vi "setSerializedData.vi"(0 "reference":refnum<class "CallNode.lvclass">, 1 "parent":refnum<class "AbstractNode.lvclass">, 2 "children":refnum<class "AbstractNode.lvclass">[](array[class]), 3 "xmlOut":string, 5 "error in (no error)":errorcluster) -> (14 "reference out":refnum<class "CallNode.lvclass">, 19 "error out":errorcluster)   [LabVIEW 2014, in "CallNode.lvclass"]
doc: "setSerializedData"
uses:
  <resource>/Framework/Providers/Open_GDS/UML/CallNode_class/CallNode.lvclass
  <resource>/Framework/Providers/Open_GDS/UML/AbstractNode_class/AbstractNode.lvclass
  <resource>/Framework/Providers/Open_GDS/UML/General/Rectangle/Rectangle Rectangle2D.ctl
  <resource>/Framework/Providers/Open_GDS/UML/RectangularNode_class/RectangularNode.lvclass
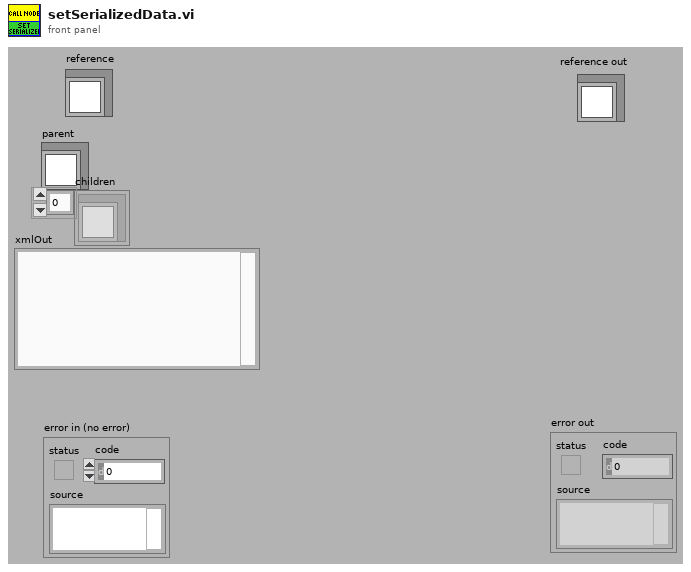
[diagram p1: front panel]
types:
  T1 = typedef "Rectangle Rectangle2D.ctl" = cluster{"x":dbl, "y":dbl, "width":dbl, "height":dbl}
  T2 = cluster{"Base class":cluster{"Base class":cluster{"parent":refnum<k1>, "children":refnum<k1>[]}, "bounds":T1}, "objectCallNodeRef":refnum<k1>, "signaled":bool, "openBottom":bool, "DEFAULT_WIDTH":i32, "DEFAULT_HEIGHT":i32, "CALL_YGAP":i32}
  T3 = typedef "RectangularNode.lvclass/ObjectAttributes.ctl" = cluster{"bounds":T1}
  T4 = typedef "AbstractNode.lvclass/ObjectAttributes.ctl" = cluster{"parent":refnum<class "AbstractNode.lvclass">, "children":refnum<class "AbstractNode.lvclass">[], "Hidden":bool}
  T5 = typedef "CallNode.lvclass/ObjectAttributes.ctl" = cluster{"objectCallNodeRef":refnum<class "AbstractNode.lvclass">, "signaled":bool, "openBottom":bool, "DEFAULT_WIDTH":i32, "DEFAULT_HEIGHT":i32, "CALL_YGAP":i32}
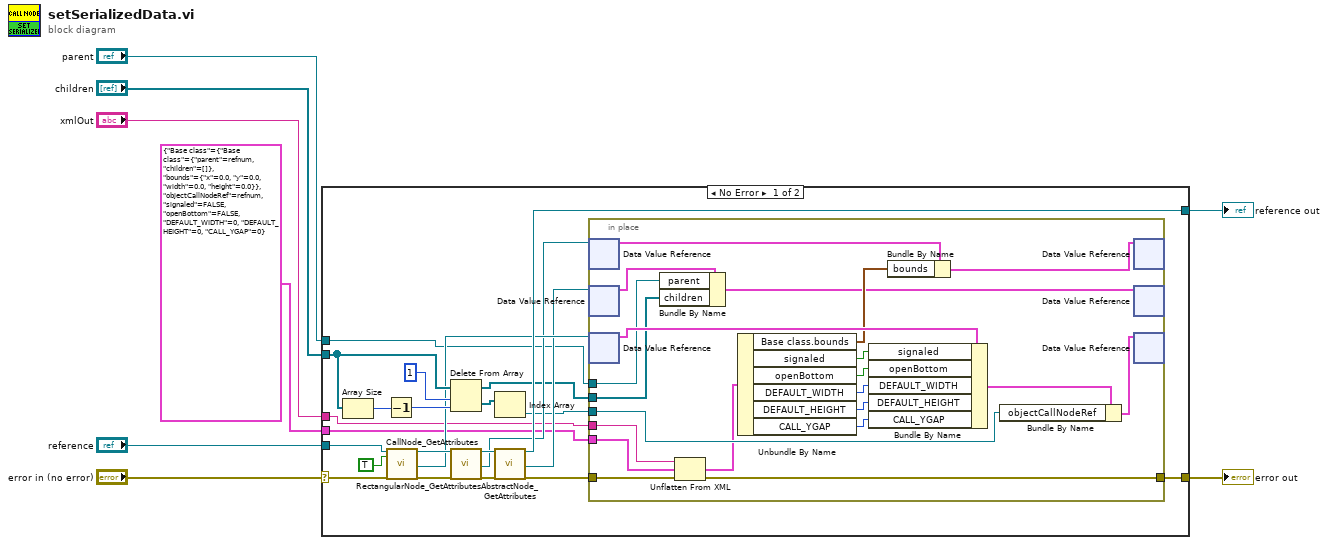
[diagram p0: block diagram]
diagram:
  n1 = case shown="No Error" "error in (no error)" {
    selector: "error in (no error)" -> [w30 w53]
    tunnel: "reference" -> [w31 w54]
    tunnel: [w29 w53] -> w6
    tunnel: [w28 w54] -> w5
    tunnel: "xmlOut" -> [w11 _]
    tunnel: "parent" -> [w10 _]
    tunnel: "children" -> [w24 _]
    tunnel: T2 {"Base class"={"Base class"={"parent"=refnum, "children"=[]}, "bounds"={"x"=0.0, "y"=0.0, "width"=0.0, "height"=0.0}}, "objectCallNodeRef"=refnum, "signaled"=FALSE, "openBottom"=FALSE, "DEFAULT_WIDTH"=0, "DEFAULT_HEIGHT"=0, "CALL_YGAP"=0} ("Attributes") -> [w12 _]
    frame No Error {
      n2 = Array Size(array=w24) -> (size(s)=w26:i32)
      n3 = Decrement(x=w26) -> (x-1=w27:i32)
      n4 = call <resource>:"CallNode_GetAttributes.vi"("reference in"=w31, "OnlyGetDvrReference(False)"=TRUE, "error in (no error)"=w30) -> ("reference out"=w21:refnum<class "CallNode.lvclass">, "DataRef"=w17:refnum<data-value>, "error out"=w20:errorcluster)  [unwired: 13 in, 1 out]
      n5 = Delete From Array(array=w24, length=1, index=w27) -> (deleted portion=w23:refnum<class "AbstractNode.lvclass">[], array with subset deleted=w9:refnum<class "AbstractNode.lvclass">[])
      n6 = call <resource>:"RectangularNode_GetAttributes.vi"("reference in"=w21, "error in (no error)"=w20) -> ("reference out"=w19:refnum<class "CallNode.lvclass">, "DataRef"=w16:refnum<data-value>, "error out"=w18:errorcluster)  [unwired: 14 in, 1 out]
      n7 = Index Array(array=w23) -> (element=w14:refnum<class "AbstractNode.lvclass">)  [unwired: 1 in]
      n8 = call <resource>:"AbstractNode_GetAttributes.vi"("reference in"=w19, "error in (no error)"=w18) -> ("reference out"=w28:refnum<class "CallNode.lvclass">, "DataRef"=w15:refnum<data-value>, "error out"=w13:errorcluster)  [unwired: 14 in, 1 out]
      n9 = in-place {
        in-place-border: w14 -> [w45]
        in-place-border: w13 -> [w41]
        in-place-border: w12 -> [w40]
        in-place-border: w11 -> [w39]
        in-place-border: [w38] -> w29
        in-place-border: w10 -> [w35]
        in-place-border: w9 -> [w34]
        n10 = in-place-dvr #1(w16) -> (w37:T3)  [unwired: 1 out]
        n11 = in-place-dvr #2(w15) -> (w36:T4)  [unwired: 1 out]
        n12 = in-place-dvr #3(w17) -> (w52:T5)  [unwired: 1 out]
        n13 = Bundle By Name(cluster=w36, "parent"=w35, "children"=w34) -> (w32:T4)
        n14 = Unflatten From XML(xml string=w39, type=w40, error in (no error)=w41) -> (value=w43:T2, error out=w38:errorcluster)
        n15 = Unbundle By Name(w43) -> ("Base class.bounds"=w42:T1, "signaled"=w51:bool, "openBottom"=w50:bool, "DEFAULT_WIDTH"=w49:i32, "DEFAULT_HEIGHT"=w48:i32, "CALL_YGAP"=w47:i32)
        n16 = Bundle By Name(cluster=w52, "signaled"=w51, "openBottom"=w50, "DEFAULT_WIDTH"=w49, "DEFAULT_HEIGHT"=w48, "CALL_YGAP"=w47) -> (w46:T5)
        n17 = Bundle By Name(cluster=w37, "bounds"=w42) -> (w33:T3)
        n18 = Bundle By Name(cluster=w46, "objectCallNodeRef"=w45) -> (w44:T5)
        n19 = in-place-dvr #1(w33) -> ()  [unwired: 2 out]
        n20 = in-place-dvr #2(w32) -> ()  [unwired: 2 out]
        n21 = in-place-dvr #3(w44) -> ()  [unwired: 2 out]
      }
    }
    frame Error {
    }
  }
  "reference out" <- w5
  "error out" <- w6
